vi "test_check engine status.vi"() -> (0 "pass 4":bool, 1 "pass 3":bool, 2 "pass 2":bool, 3 "pass":bool)   [LabVIEW 2014]
uses:
  <vilib>/NI/Module Execution Interface/Engine Runtime/Execution States.ctl
  <vilib>/NI/Module Execution Interface/Engine Runtime/Fault.ctl
  <vilib>/NI/Tag Bus Module Framework/runtime/error classification.ctl
  <vilib>/NI/Tag Bus Module Framework/runtime/TBM module execution interface.lvclass
  <vilib>/NI/Module Execution Interface/Engine Runtime/Engine Runtime Interface.lvclass
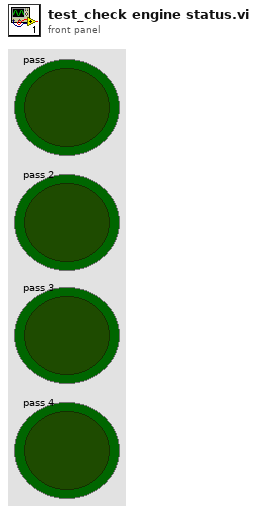
[diagram p1: front panel]
types:
  T1 = typedef "Engine Runtime Interface.lvclass/Execution States.ctl" = enum16{"Init", "Pre-Operational", "Safe-Operational", "Operational", "Stopped"}
  T2 = typedef "Engine Runtime Interface.lvclass/Fault.ctl" = cluster{"code":i32, "error classification":T3, "Source GUID":string, "first reported time":timestamp, "number reported":u32, "last reported time":timestamp}
  T3 = typedef "TBM module execution interface.lvclass/error classification.ctl" = enum16{"unknown", "none", "trivial", "recoverable", "critical"}
  T4 = cluster{"Engine State":T1, "Fault Buffer":T2[], "Engine Error":errorcluster}[]
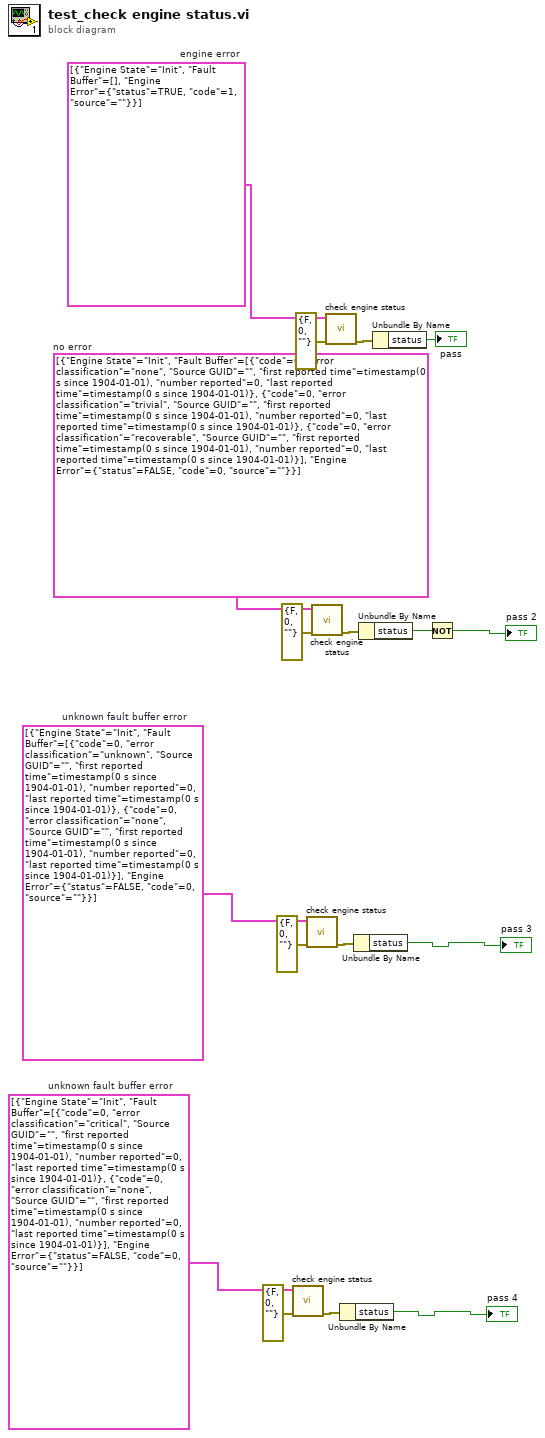
[diagram p0: block diagram]
diagram:
  w3 = T4 [{"Engine State"=enum."Init", "Fault Buffer"=[{"code"=0, "error classification"=enum."none", "Source GUID"="", "first reported time"=timestamp(0 s since 1904-01-01), "number reported"=0, "last reported time"=timestamp(0 s since 1904-01-01)}, {"code"=0, "error classification"=enum."trivial", "Source GUID"="", "first reported time"=timestamp(0 s since 1904-01-01), "number reported"=0, "last reported time"=timestamp(0 s since 1904-01-01)}, {"code"=0, "error classification"=enum."recoverable", "Source GUID"="", "first reported time"=timestamp(0 s since 1904-01-01), "number reported"=0, "last reported time"=timestamp(0 s since 1904-01-01)}], "Engine Error"={"status"=FALSE, "code"=0, "source"=""}}]  # no error
  w9 = T4 [{"Engine State"=enum."Init", "Fault Buffer"=[], "Engine Error"={"status"=TRUE, "code"=1, "source"=""}}]  # engine error
  w10 = T4 [{"Engine State"=enum."Init", "Fault Buffer"=[{"code"=0, "error classification"=enum."critical", "Source GUID"="", "first reported time"=timestamp(0 s since 1904-01-01), "number reported"=0, "last reported time"=timestamp(0 s since 1904-01-01)}, {"code"=0, "error classification"=enum."none", "Source GUID"="", "first reported time"=timestamp(0 s since 1904-01-01), "number reported"=0, "last reported time"=timestamp(0 s since 1904-01-01)}], "Engine Error"={"status"=FALSE, "code"=0, "source"=""}}]  # unknown fault buffer error
  w17 = T4 [{"Engine State"=enum."Init", "Fault Buffer"=[{"code"=0, "error classification"=enum."unknown", "Source GUID"="", "first reported time"=timestamp(0 s since 1904-01-01), "number reported"=0, "last reported time"=timestamp(0 s since 1904-01-01)}, {"code"=0, "error classification"=enum."none", "Source GUID"="", "first reported time"=timestamp(0 s since 1904-01-01), "number reported"=0, "last reported time"=timestamp(0 s since 1904-01-01)}], "Engine Error"={"status"=FALSE, "code"=0, "source"=""}}]  # unknown fault buffer error
  n1 = call "check engine status.vi"("error in (no error)"=errorcluster {"status"=FALSE, "code"=0, "source"=""}, "engine status"=w10) -> ("error out"=w12:errorcluster)  [unwired: 8 in, 1 out]
  n2 = call "check engine status.vi"("error in (no error)"=errorcluster {"status"=FALSE, "code"=0, "source"=""}, "engine status"=w17) -> ("error out"=w15:errorcluster)  [unwired: 8 in, 1 out]
  n3 = call "check engine status.vi"("error in (no error)"=errorcluster {"status"=FALSE, "code"=0, "source"=""}, "engine status"=w3) -> ("error out"=w5:errorcluster)  [unwired: 8 in, 1 out]
  n4 = call "check engine status.vi"("error in (no error)"=errorcluster {"status"=FALSE, "code"=0, "source"=""}, "engine status"=w9) -> ("error out"=w7:errorcluster)  [unwired: 8 in, 1 out]
  n5 = Unbundle By Name(w12) -> ("status"=→"pass 4":bool)
  n6 = Unbundle By Name(w15) -> ("status"=→"pass 3":bool)
  n7 = Unbundle By Name(w5) -> ("status"=w2:bool)
  n8 = Unbundle By Name(w7) -> ("status"=→"pass":bool)
  n9 = Not(x=w2) -> (.not. x?=→"pass 2":bool)
